vi "textColor.vi"(11 "디지털 입력":refnum<vi>) -> ()   [LabVIEW 2019]
uses:
  <vilib>/Utility/miscctls.llb/LVSelectionTypeDef.ctl
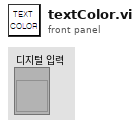
[diagram p1: front panel]
types:
  T1 = typedef "LVSelectionTypeDef.ctl" = cluster{"Selection Start":u32, "Selection End":u32}
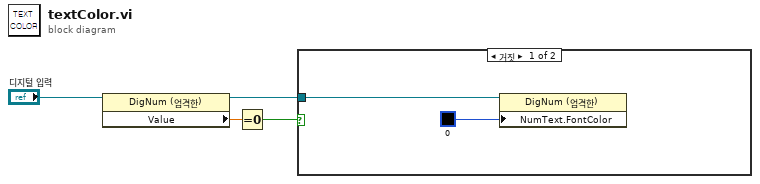
[diagram p0: block diagram]
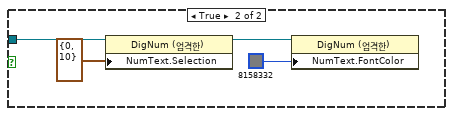
[diagram p2: hidden frame]
diagram:
  n1 = property on="프로퍼티 노드" class="DigNum (엄격한)"(reference="디지털 입력") -> (reference out=w3:refnum<vi>, "Value"=w2:dbl)  [unwired: 1 in, 1 out]
  n2 = Equal To 0?(x=w2) -> (x = 0?=w1:bool)
  n3 = case shown="거짓" w1 {
    tunnel: w3 -> [w5 w8]
    frame False {
      n4 = property on="프로퍼티 노드" class="DigNum (엄격한)"(reference=w5, "NumText.FontColor"=u32 0 ("숫자형 텍스트.폰트:색")) -> ()  [unwired: 1 in, 2 out]
    }
    frame True {
      n5 = property on="프로퍼티 노드" class="DigNum (엄격한)"(reference=w8, "NumText.Selection"=T1 {"Selection Start"=0, "Selection End"=10} ("숫자형 텍스트.선택")) -> (reference out=w7:refnum<vi>)  [unwired: 1 in, 1 out]
      n6 = property on="프로퍼티 노드" class="DigNum (엄격한)"(reference=w7, "NumText.FontColor"=u32 8158332 ("숫자형 텍스트.폰트:색")) -> ()  [unwired: 1 in, 2 out]
    }
  }
